vi "Motion Control Module.vi"(5 "Set/Get":T1=enum."Get", 7 "Action":T3=enum."Stop", 8 "Error In":errorcluster, 10 "LTS Reference":refnum<k24>(container), 11 "Cluster":T2={"Device SN"="45876539", "Is.Connected?"=FALSE, "Is.Enabled?"=FALSE, "Position"=0.0, "AccelerationMaximum"=0.0, "VelocityMaximum"=0.0, "Acceleration"=0.0, "Velocity"=0.0, "waitTimeout (ms)"=0}) -> (0 "Error Out":errorcluster, 2 "LTS Reference Out":refnum<k24>(container), 3 "Cluster":T2={"Device SN"="45876539", "Is.Connected?"=FALSE, "Is.Enabled?"=FALSE, "Position"=0.0, "AccelerationMaximum"=0.0, "VelocityMaximum"=0.0, "Acceleration"=0.0, "Velocity"=0.0, "waitTimeout (ms)"=0})   [LabVIEW 2014]
uses:
  C:/Projects/Serial Sectioning OCT - TortoiseGIT/SerialSectOCT/Software/Test Code/Thorlabs.MotionControl.Controls.dll
  Thorlabs.MotionControl.Controls.dll
  Ctrls/Translation Stage Cluster.ctl
  Ctrls/Motion Translation Module Control.ctl
  General/Controls/Set Get Controls.ctl
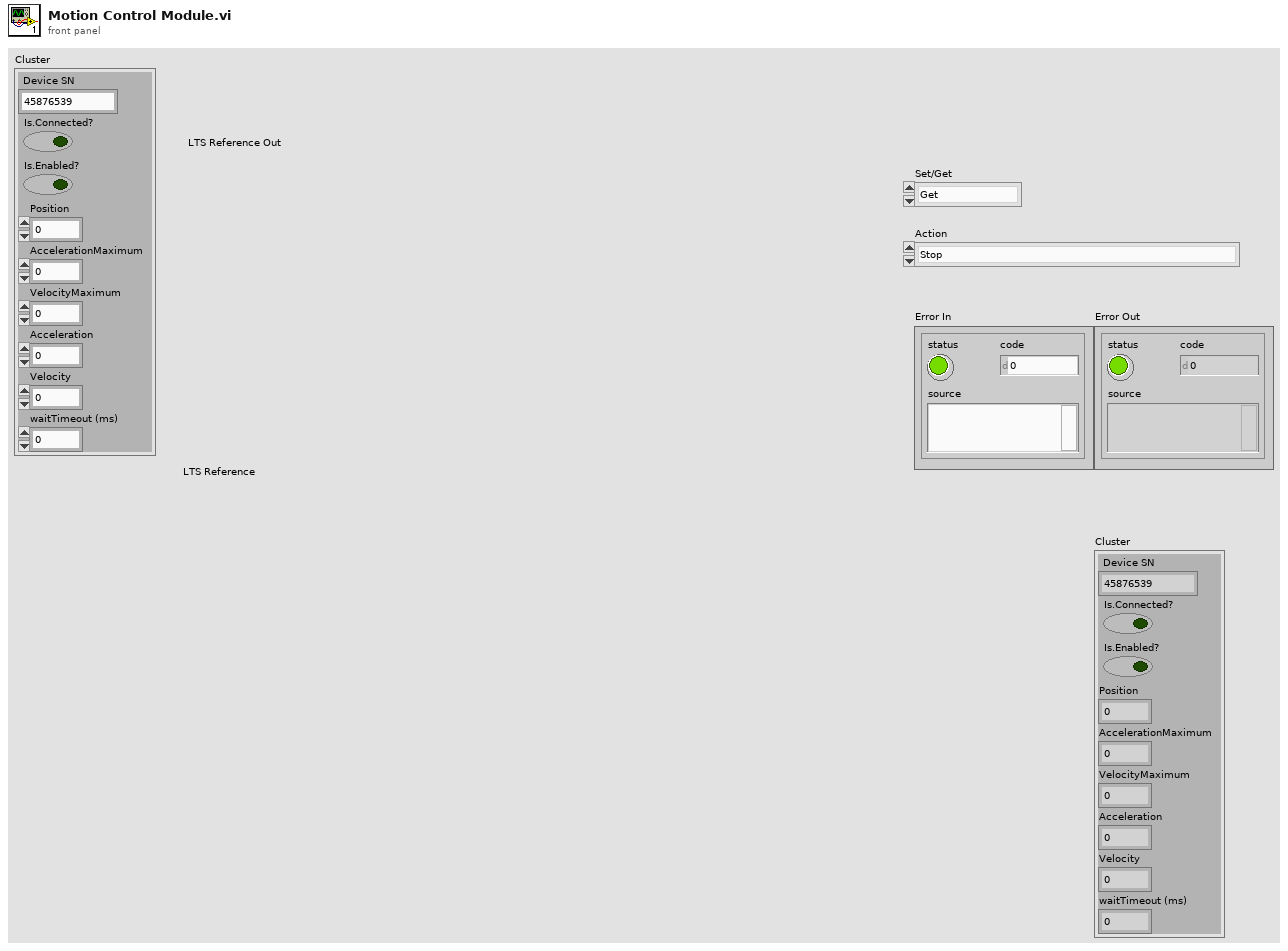
[diagram p1: front panel]
types:
  T1 = typedef "Set Get Controls.ctl" = enum16{"Set", "Get"}
  T2 = typedef "Translation Stage Cluster.ctl" = cluster{"Device SN":string, "Is.Connected?":bool, "Is.Enabled?":bool, "Position":dbl, "AccelerationMaximum":dbl, "VelocityMaximum":dbl, "Acceleration":dbl, "Velocity":dbl, "waitTimeout (ms)":i32}
  T3 = typedef "Motion Translation Module Control.ctl" = enum16{"Init", "Home", "Configure", "Velocity/Accel", "Position", "Jog", "Stop", "Uninit"}
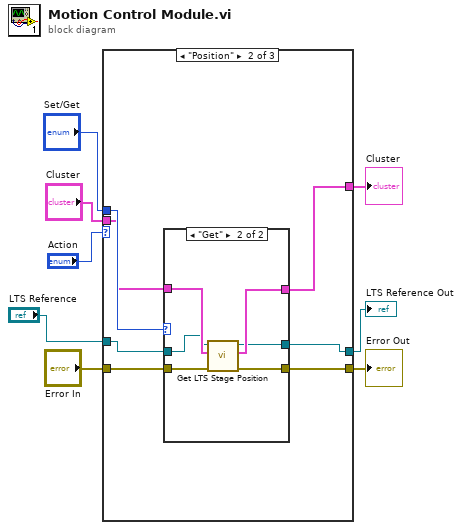
[diagram p0: block diagram]
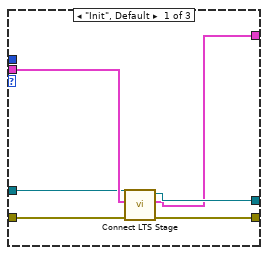
[diagram p2: hidden frame]
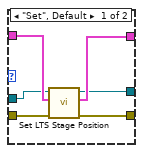
[diagram p3: hidden frame]
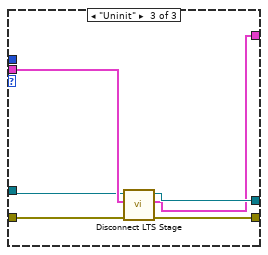
[diagram p4: hidden frame]
diagram:
  n1 = case shown="\"Position\"" "Action" {
    tunnel: "Set/Get" -> [_ w21 _]
    tunnel: "Cluster" -> [w12 w18 w36]
    tunnel: "Error In" -> [w14 w20 w39]
    tunnel: [w11 w16 w37] -> w4
    tunnel: [w13 w19 w38] -> w3
    tunnel: [w10 w17 w35] -> w2
    tunnel: "LTS Reference" -> [w9 w15 w34]
    frame "Init", Default {
      n2 = call "Connect LTS Stage.vi"("error in (no error)"=w14, "Cluster in"=w12, "LTS Reference In"=w9) -> ("error out"=w13:errorcluster, "Cluster out"=w10:T2, "LTS Reference Out"=w11:refnum<k24>)  [unwired: 5 in, 1 out]
    }
    frame "Position" {
      n3 = case shown="\"Get\"" w21 {
        tunnel: w20 -> [w27 w33]
        tunnel: [w26 w32] -> w19
        tunnel: w18 -> [w25 w31]
        tunnel: [w24 w30] -> w17
        tunnel: w15 -> [w23 w29]
        tunnel: [w22 w28] -> w16
        frame "Set", Default {
          n4 = call "Set LTS Stage Position.vi"("error in (no error)"=w27, "Cluster in"=w25, "LTS Reference In"=w23) -> ("error out"=w26:errorcluster, "Cluster out"=w24:T2, "LTS Reference Out"=w22:refnum<k24>)  [unwired: 6 in]
        }
        frame "Get" {
          n5 = call "Get LTS Stage Position.vi"("error in (no error)"=w33, "Cluster in"=w31, "LTS Reference In"=w29) -> ("error out"=w32:errorcluster, "Cluster out"=w30:T2, "LTS Reference Out"=w28:refnum<k24>)  [unwired: 5 in, 1 out]
        }
      }
    }
    frame "Uninit" {
      n6 = call "Disconnect LTS Stage.vi"("error in (no error)"=w39, "Cluster in"=w36, "LTS Reference In"=w34) -> ("error out"=w38:errorcluster, "Cluster out"=w35:T2, "LTS Reference Out"=w37:refnum<k24>)  [unwired: 6 in]
    }
  }
  "Error Out" <- w3
  "Cluster" <- w2
  "LTS Reference Out" <- w4
